vi "Discard Menu Build Language Item.vi"() -> (3 "Menu File Item":refnum<data-value>)   [LabVIEW 2018, in "LF2R IDE.lvlib" / "LF2R IDE.lvclass"]
uses:
  LF2R IDE.lvclass
  <userlib>/_MGI/Menu Building/MenuItem/MGI_MenuItem.lvclass
  <userlib>/_MGI/Menu Building/SelectionType/RadioSelection/MGI_RadioSelection.lvclass
  C:/Program Files (x86)/National Instruments/LabVIEW 2018/user.lib/_MGI/Menu Building/SelectionType/MGI_SelectionType.lvclass
  <userlib>/_MGI/Menu Building/MenuItem/MenuItem.vi
  <userlib>/_MGI/Menu Building/SelectionType/RadioSelection/RadioSelection.vi
  <userlib>/_MGI/Menu Building/MenuItem/Write Sub-Menus.vi
  <userlib>/_MGI/Menu Building/SelectionType/MGI_SelectionType.lvclass
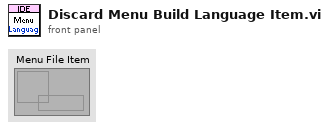
[diagram p1: front panel]
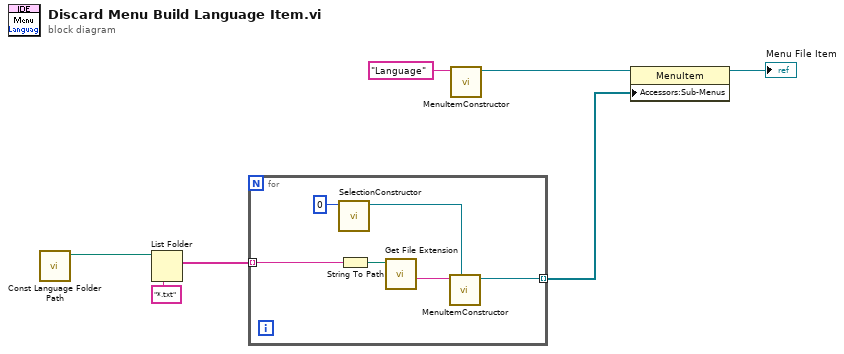
[diagram p0: block diagram]
diagram:
  n1 = call "Const Language Folder Path.vi"() -> ("Language Folder Path"=w4:path)  [unwired: 11 in]
  n2 = List Folder(path=w4, pattern="*.txt") -> (filenames=w2:string[])  [unwired: 2 in, 3 out]
  n3 = for {
    tunnel: w2 -> [w12] mode=indexing
    tunnel: [w13] -> w1 mode=indexing
    n4 = call-poly <userlib>:"SelectionConstructor.vi"("Group"=u8 0) -> ("RadioSelection out"=w9:refnum<class "MGI_RadioSelection.lvclass">)  [unwired: 9 in, 1 out]
    n5 = String To Path(string=w12) -> (path=w11:path)
    n6 = call <vilib>:"Get File Extension.vi"("file"=w11) -> ("filename without extension"=w10:string)  [unwired: 6 in, 4 out]
    n7 = call-poly <userlib>:"MenuItemConstructor.vi"("Selection Type"=w9, "Text"=w10) -> ("MenuItem"=w13:refnum<data-value>)  [unwired: 8 in, 1 out]
  }
  n8 = call-poly <userlib>:"MenuItemConstructor.vi"("Text"="Language") -> ("MenuItem"=w7:refnum<data-value>)  [unwired: 9 in, 1 out]
  n9 = property class="MenuItem"(reference=w7, "Accessors:Sub-Menus"=w1) -> (reference out=→"Menu File Item":refnum<data-value>)  [unwired: 1 in, 1 out]
